vi "Teleop One Pass.vi"() -> ()   [LabVIEW 2013]
uses:
  Drive Train/Drive Train Class/Drive Train Status.ctl
  Robot Actors/System Actor/System Actor Class/System Status.ctl
  Robot Actors/Command/Command Class/Command Status.ctl
  Driver Status.ctl
  XBox Controller/Xbox Controller.ctl
  Virtual Systems/XBox Controller/XBox Controller Class/Joystick.ctl
  Drive Train/Drive Train Messages/Write Drive Train Status Ref Msg/Write Drive Train Status Ref Msg.lvclass/Write Drive Train Status Ref Msg.ctl
  <vilib>/ActorFramework/Message Enqueuer/Message Enqueuer.lvclass/Message Enqueuer.ctl
  Robot Actors/System Actor/System Actor Messages/Write System Status Ref Msg/Write System Status Ref Msg.lvclass/Write System Status Ref Msg.ctl
  Driver Messages/Write Driver Status Ref Msg/Write Driver Status Ref Msg.lvclass/Write Driver Status Ref Msg.ctl
  <vilib>/ActorFramework/Message Enqueuer/Enqueue.vi
  Virtual Robot/Robot Global.vi
  <vilib>/ActorFramework/Message Priority Queue/Priority Enqueue.vi
  Drive Train/Drive Train Messages/Write Drive Train Status Ref Msg/Write Drive Train Status Ref Msg.lvclass
  Robot Actors/System Actor/System Actor Messages/Write System Status Ref Msg/Write System Status Ref Msg.lvclass
  Driver Messages/Write Driver Status Ref Msg/Write Driver Status Ref Msg.lvclass
  Drive Train/Drive Train Class/Drive Train.lvclass
  Robot Actors/Command/Command Class/Command.lvclass
  Robot Actors/System Actor/System Actor Class/System Actor.lvclass
  XBox Controller/XBox Controller Class/Xbox Controller.lvlib
  Driver.lvclass
panel:
  in  "Driver - System Status":T1
  in  "Driver Status":T3 {"Current Xbox Controller"."Right Joystick"."Right" min=-1.0 max=1.0 step=0.1 scale=-1.0..1.0; "Current Xbox Controller"."Right Joystick"."Forward" min=-1.0 max=1.0 step=0.1 scale=-1.0..1.0; "Current Xbox Controller"."Left Joystick"."Right" min=-1.0 max=1.0 step=0.1 scale=-1.0..1.0; "Current Xbox Controller"."Left Joystick"."Forward" min=-1.0 max=1.0 step=0.1 scale=-1.0..1.0}
  in  "Drive Train - System Status":T1
  in  "Drive Train Status":T6 {"Right Power Setpoint" min=-1.0 max=1.0 step=0.1 scale=-1.0..1.0; "Left Power Setpoint" min=-1.0 max=1.0 step=0.1 scale=-1.0..1.0; "Right Power" min=-1.0 max=1.0 step=0.1 scale=-1.0..1.0; "Left Power" min=-1.0 max=1.0 step=0.1 scale=-1.0..1.0}
  in  "Fire One Pass":bool
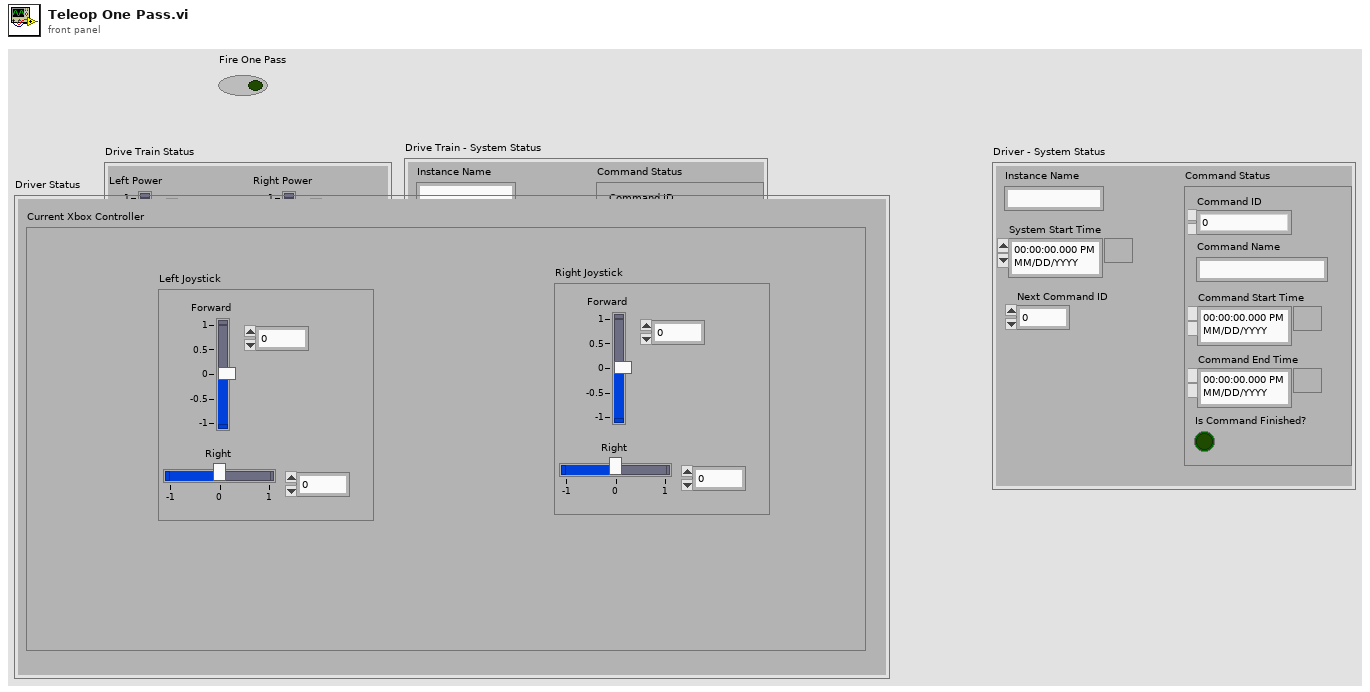
[diagram p1: front panel]
types:
  T1 = typedef "Robot Actors.lvlib/System Actor.lvlib/System Actor.lvclass/System Status.ctl" = cluster{"Instance Name":string, "Command Status":T2, "System Start Time":timestamp, "Next Command ID":dbl}
  T2 = typedef "Robot Actors.lvlib/Command.lvlib/Command.lvclass/Command Status.ctl" = cluster{"Command Name":string, "Command Start Time":timestamp, "Command End Time":timestamp, "Is Command Finished?":bool, "Command ID":dbl}
  T3 = typedef "Logical Systems.lvlib/Driver.lvlib/Driver.lvclass/Driver Status.ctl" = cluster{"Current Xbox Controller":T4}
  T4 = typedef "Logical Systems.lvlib/Xbox Controller.lvlib/Xbox Controller.ctl" = cluster{"Left Joystick":T5, "Right Joystick":T5}
  T5 = typedef "Logical Systems.lvlib/Xbox Controller.lvlib/Joystick.ctl" = cluster{"Forward":dbl, "Right":dbl}
  T6 = typedef "Logical Systems.lvlib/Drive Train.lvlib/Drive Train.lvclass/Drive Train Status.ctl" = cluster{"Left Power":dbl, "Right Power":dbl, "Left Power Setpoint":dbl, "Right Power Setpoint":dbl}
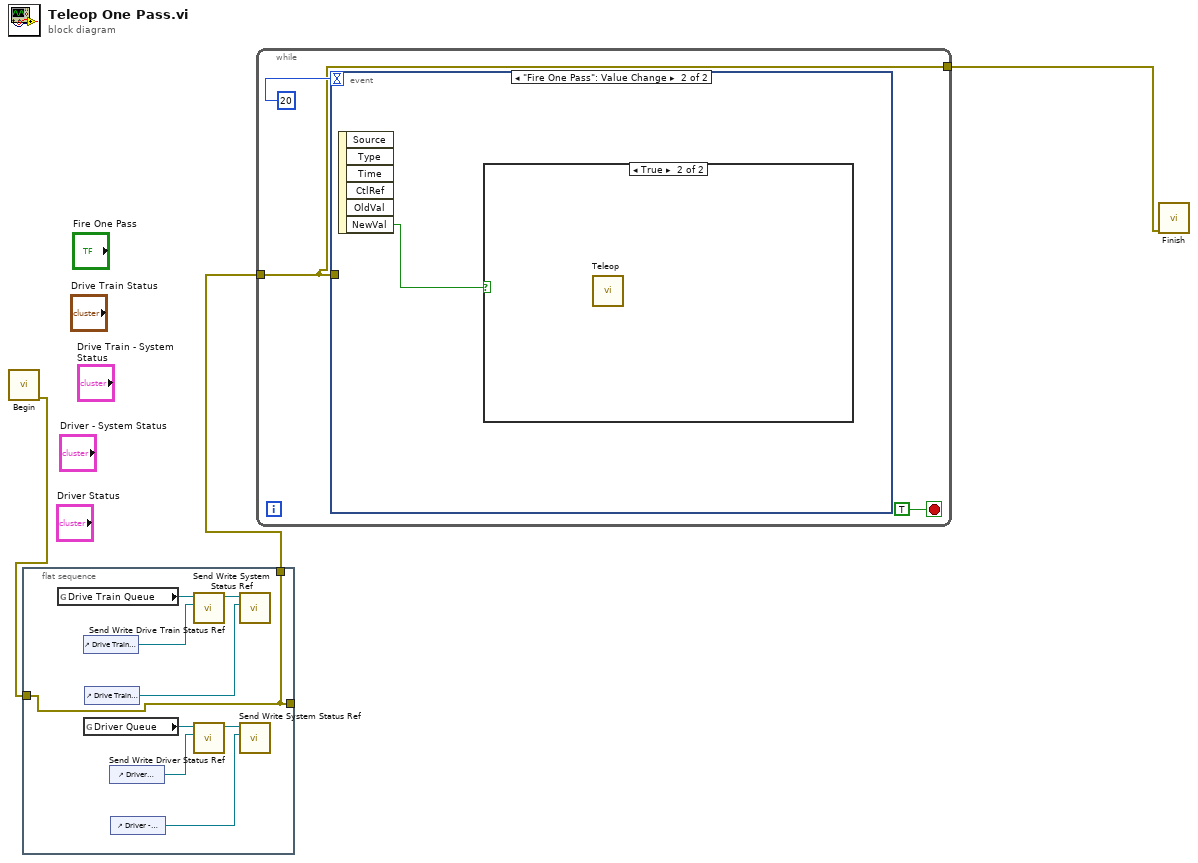
[diagram p0: block diagram]
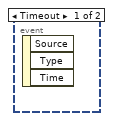
[diagram p2: hidden frame]
diagram:
  n1 = call "Begin.vi"() -> ("error out"=w3:errorcluster)  [unwired: 11 in]
  n2 = flat-sequence {
    tunnel: w3 -> [w4]
    tunnel: [w4] -> _
    tunnel: [w4] -> w2
    frame #0 {
      n3 = global read "Robot Global.vi" "Drive Train Queue"() -> (w12:refnum<class "Message Enqueuer.lvclass">)
      n4 = control-ref of="Drive Train Status"() -> (w11:refnum<vi>)
      n5 = global read "Robot Global.vi" "Driver Queue"() -> (w8:refnum<class "Message Enqueuer.lvclass">)
      n6 = control-ref of="Drive Train - System Status"() -> (w9:refnum<vi>)
      n7 = control-ref of="Driver Status"() -> (w7:refnum<vi>)
      n8 = control-ref of="Driver - System Status"() -> (w5:refnum<vi>)
      n9 = call "Send Write Drive Train Status Ref.vi"("Drive Train Status Ref"=w11, "Message Enqueuer"=w12) -> ("Message Enqueuer out"=w10:refnum<class "Message Enqueuer.lvclass">)  [unwired: 8 in, 1 out]
      n10 = call "Send Write Driver Status Ref.vi"("Driver Status Ref"=w7, "Message Enqueuer"=w8) -> ("Message Enqueuer out"=w6:refnum<class "Message Enqueuer.lvclass">)  [unwired: 8 in, 1 out]
      n11 = call "Send Write System Status Ref.vi"("System Status Ref"=w9, "Message Enqueuer"=w10) -> ()  [unwired: 8 in, 2 out]
      n12 = call "Send Write System Status Ref.vi"("System Status Ref"=w5, "Message Enqueuer"=w6) -> ()  [unwired: 8 in, 2 out]
    }
  }
  n13 = while {
    tunnel: w2 -> [w13]
    tunnel: [w13] -> w1
    stop <- TRUE stop-if-true
    n14 = event shown="[1] \"Fire One Pass\": Value Change" {
      selector: _ -> [_ _]
      dyn-events: _ -> [_ _]
      timeout: 20 -> [_ _]
      tunnel: w13 -> [_ _]
      event Timeout {
        n15 = event-data() -> ()  [unwired: 1 in, 3 out]
      }
      event "Fire One Pass": Value Change {
        n16 = event-data() -> ("NewVal"=w16:bool)  [unwired: 1 in, 5 out]
        n17 = case shown="True" w16 {
          frame False {
          }
          frame True {
            n18 = call "Teleop.vi"() -> ()  [unwired: 12 in]
          }
        }
      }
    }
  }
  n19 = call "Finish.vi"("error in (no error)"=w1) -> ()  [unwired: 11 in]
